vi "RD Digital Out Enable Set.vi"(8 "error in (no error)":errorcluster caption="错误输入（无错误）", 10 "chs":u32, 11 "handle":u64) -> (0 "error out":errorcluster caption="错误输出", 2 "function return":i32, 3 "handle out":u64)   [LabVIEW 2018, in "InstrumentsPlayground.lvlib"]
doc: "CLIFFAPI int CliffDigitalOutEnableSet(FT_HANDLE handle, uint chs);\nchs:0XFFFF :: DIO 16->1 each switch ex.0x0001for ch1 output enable. 0xFFFF for all DIO output enable."
uses:
  InstrumentsPlayground.lvlib
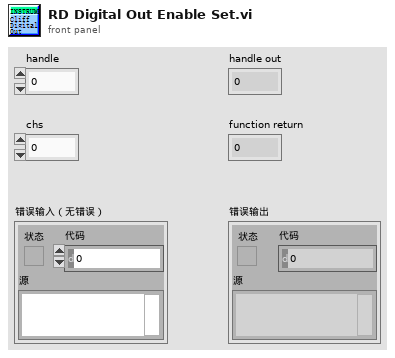
[diagram p1: front panel]
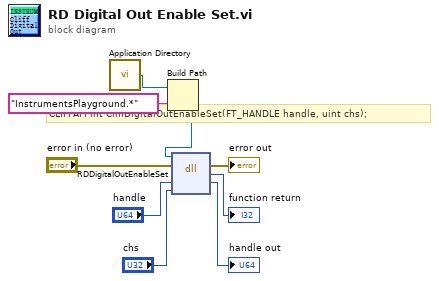
[diagram p0: block diagram]
diagram:
  # "CLIFFAPI int CliffDigitalOutEnableSet(FT_HANDLE handle, uint chs);"
  n1 = call <vilib>:"Application Directory.vi"() -> ("Application Directory"=w2:path)
  n2 = Build Path(base path=w2, name or relative path="InstrumentsPlayground.*" ("名称或相对路径")) -> (appended path=w1:path)
  n3 = dll-call lib="E:/work/YZCourse_Xtext/Cliff/API/LabVIEW lib/InstrumentsPlayground.*" fn="RDDigitalOutEnableSet"(path in=w1, error in="error in (no error)", "handle"="handle", "chs"="chs") -> (error out=→"error out":errorcluster, "返回类型"=→"function return":i32, "handle"=→"handle out":u64)  [unwired: 2 in, 1 out]
